vi "Control.vi"() -> ()   [LabVIEW 2021]
uses:
  <vilib>/Utility/error.llb/DialogType.ctl
  <vilib>/DAQmx/write.llb/DAQmx Write (Digital U8 1Chan 1Samp).vi
  <vilib>/DAQmx/read.llb/DAQmx Read (Analog 1D Wfm NChan 1Samp).vi
  <vilib>/DAQmx/write.llb/DAQmx Write (Analog DBL 1Chan 1Samp).vi
  <vilib>/DAQmx/create/channels.llb/DAQmx Create Channel (AO-Voltage-Basic).vi
  <vilib>/DAQmx/create/channels.llb/DAQmx Create Channel (AI-Voltage-Basic).vi
  <vilib>/DAQmx/create/channels.llb/DAQmx Create Channel (DO-Digital Output).vi
  <vilib>/DAQmx/miscellaneous.llb/DAQmx Fill In Error Info.vi
  <vilib>/Utility/file.llb/Read Delimited Spreadsheet (string).vi
  <vilib>/addons/control/pid/pid.llb/PID (DBL).vi
  <vilib>/Utility/file.llb/Write Delimited Spreadsheet (string).vi
  <vilib>/Analysis/NI_AALBase.lvlib
  <vilib>/addons/control/pid/NI_PID_pid.lvlib
panel:
  out "Duración real":dbl
  out "Señal de error":waveform(dbl)(graph)
  out "Señal de control":waveform(dbl)(graph)
  in  "Offset":dbl=0.0001012992 format="%.6e"
  in  "Amplitud":dbl=0.01 format="%.6e"
  out "Señal de realimentación":waveform(dbl)(graph)
  in  "n":dbl=-0.05522872 format="%.6e"
  in  "m":dbl=0.01426491 format="%_6e"
  out "Archivo a generar":string
  out "Experimento Nº":i16=1
  in  "Grabar":bool
  out "Salida sensor de curvatura":waveform(dbl)(graph)
  out "Salida sensor de presión":waveform(dbl)(graph)
  in  "Válvula":bool
  in  "stop":bool
  out "Consigna":waveform(dbl)(graph)
  in  "Comenzar":bool
  in  "Ciclo de trabajo":dbl=1.0 format="%#_2f"
  in  "f1":dbl=10.0 format="%.2f"
  in  "Info. muestreo":cluster{"Fs":dbl, "t":dbl}={"Fs"=100.0, "t"=10.0} {"Fs" format="%.2p"}
  in  "Fase":dbl format="%.2f"
  in  "f0":dbl=10.0 format="%.2f"
  in  "Señal":u16(ring)=2 items=["Senoidal", "Chirp", "Escalón"]
  out "Salida regulador de presión":waveform(dbl)(graph)
  in  "Parar":bool
  # "+"
  # "ACTUADOR"
  # "-"
  # "Calibración sensor"
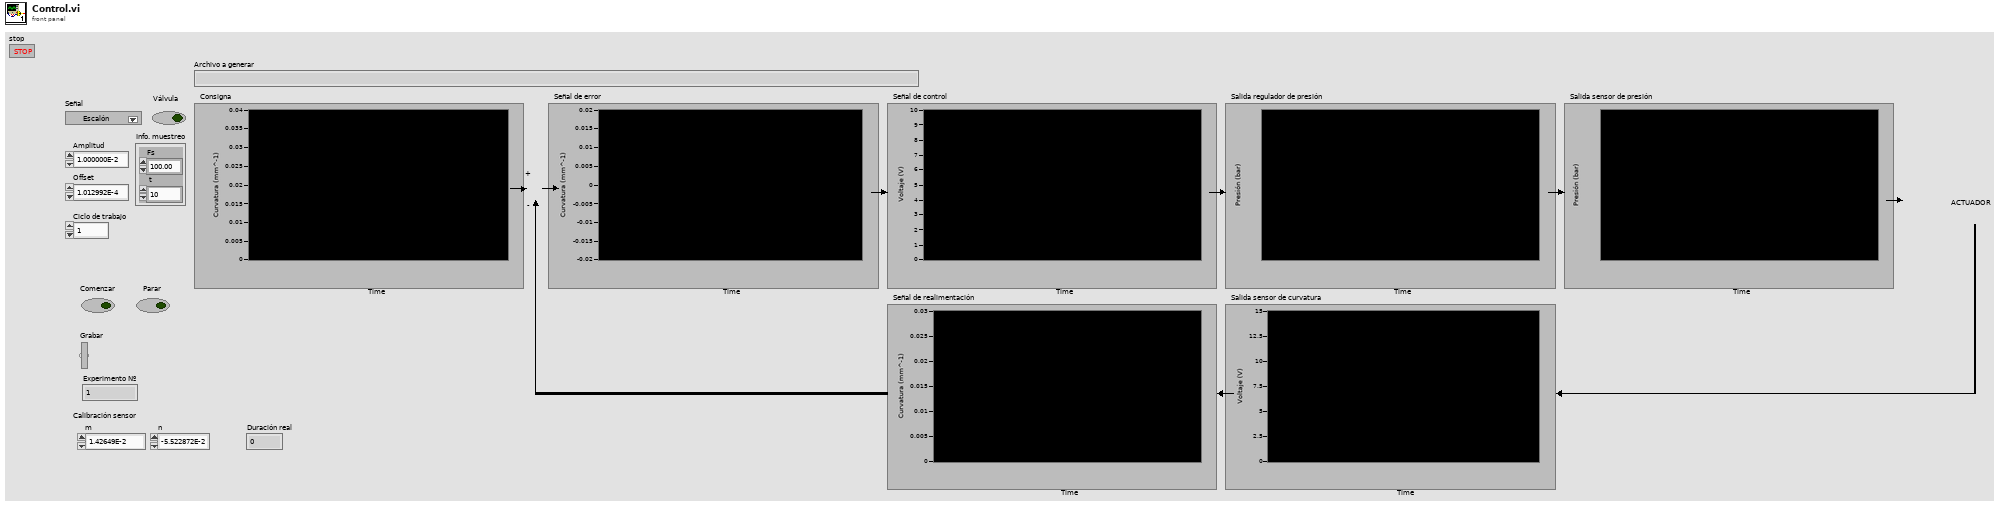
[diagram p1: front panel]
types:
  T1 = cluster{"proportional gain (Kc)":dbl, "integral time (Ti, min)":dbl, "derivative time (Td, min)":dbl}
  T2 = typedef "DialogType.ctl" = u16
  T3 = typedef "NI_Matrix.lvlib/RealMatrix.ctl" = dbl[][]
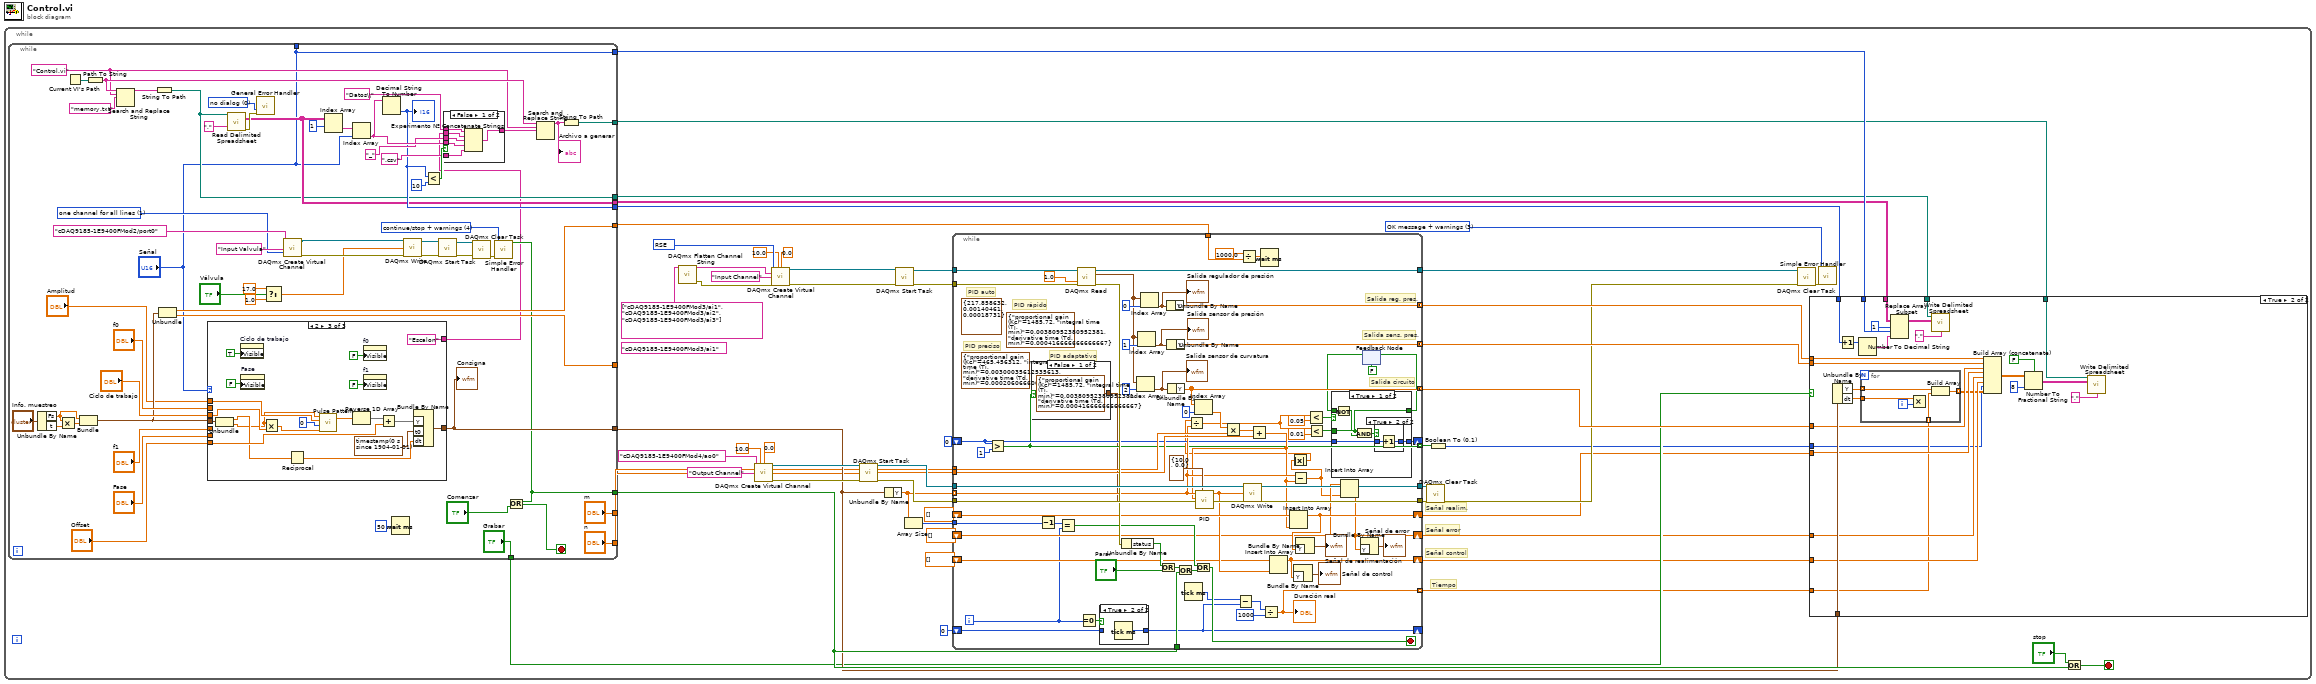
[diagram p0: block diagram]
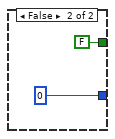
[diagram p4: hidden frame]
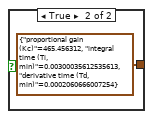
[diagram p5: hidden frame]
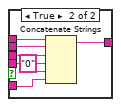
[diagram p7: hidden frame]
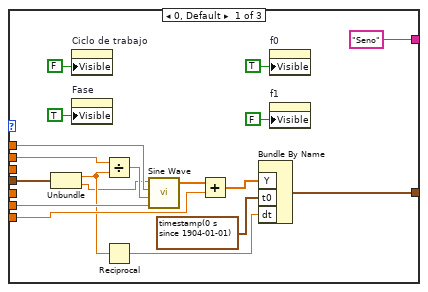
[diagram p8: hidden frame]
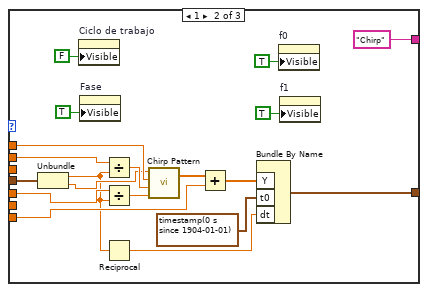
[diagram p9: hidden frame]
diagram:
  n1 = while {
    stop <- w47 stop-if-true
    w49 = T2 3 items=["no dialog", "OK message", "continue or stop message", "OK message + warnings", "continue/stop + warnings"] ("type of dialog (OK msg:1)")
    w45 = 10083 items=["Default"=-1, "RSE"=10083, "NRSE"=10078, "Differential"=10106, "Pseudodifferential"=12529] ("input terminal configuration")
    (unwired) tag "cDAQ9185-1E9400FMod3/ai1" ("physical channels")
    # "Tiempo"
    # "Señal error"
    # "Señal realim."
    # "Señal control"
    n2 = while {
      tunnel: [w222] -> w30
      tunnel: [w229] -> w32
      tunnel: [w223] -> _
      tunnel: [w203] -> w40
      tunnel: ["Señal"] -> _
      tunnel: [w184] -> w28
      tunnel: [w183] -> w27
      tunnel: [w182] -> w26
      tunnel: ["Señal"] -> w29
      tunnel: [w179] -> w25
      tunnel: ["Grabar"] -> w24
      tunnel: ["m"] -> w23
      tunnel: ["n"] -> w22
      stop <- w213 stop-if-true
      w189 = T2 0 items=["no dialog", "OK message", "continue or stop message", "OK message + warnings", "continue/stop + warnings"] ("type of dialog (OK msg:1)")
      w186 = "Control.vi" ("substring (\"\")")
      w208 = 1 items=["one channel for each line", "one channel for all lines"] ("line grouping")
      w220 = T2 4 items=["no dialog", "OK message", "continue or stop message", "OK message + warnings", "continue/stop + warnings"] ("type of dialog (OK msg:1)")
      n3 = Unbundle By Name("Info. muestreo") -> ("Fs"=w225:dbl, "t"=w227:dbl)
      n4 = Multiply(x=w225, y=w227) -> (x*y=w226:dbl)
      n5 = Current VI's Path() -> (path=w194:path)
      n6 = Bundle("Fs"=w225, w226) -> (w224:cluster{"Fs":dbl, dbl})  [unwired: 1 in]
      n7 = Path To String(path=w194) -> (string=w195:string)
      n8 = Search and Replace String(input string=w195, search string=w186, replace string="memory.txt" ("replace string (\"\")")) -> (result string=w196:string)  [unwired: 5 in, 3 out]
      n9 = String To Path(string=w196) -> (path=w182:path)
      n10 = Unbundle(w224) -> ("Fs"=w222:dbl, w223:dbl)
      n11 = case shown="2" "Señal" {
        tunnel: [w261 w273 w301] -> w229
        tunnel: "f0" -> [w259 w279 _]
        tunnel: "Amplitud" -> [w257 w283 w297]
        tunnel: "Fase" -> [w255 _ _]
        tunnel: w224 -> [w254 w272 w291]
        tunnel: "f1" -> [_ w280 _]
        tunnel: "Offset" -> [w260 w281 w293]
        tunnel: "Ciclo de trabajo" -> [_ _ w299]
        tunnel: ["Seno" "Chirp" "Escalon"] -> w180
        frame 0, Default {
          n12 = Unbundle(w254) -> ("Fs"=w253:dbl, w252:dbl)
          n13 = property on="Ciclo de trabajo" class="DigNum (strict)"("Visible"=FALSE) -> ()  [unwired: 2 in, 2 out]
          n14 = property on="Fase" class="DigNum (strict)"("Visible"=TRUE) -> ()  [unwired: 2 in, 2 out]
          n15 = Divide(x=w259, y=w253) -> (x/y=w256:dbl)
          n16 = Reciprocal(x=w253) -> (1/x=w263:dbl)
          n17 = call <vilib>:"Sine Wave.vi"("samples"=w252, "amplitude"=w257, "frequency"=w256, "phase in"=w255) -> ("sine wave"=w258:dbl[])  [unwired: 1 in, 2 out]
          n18 = Add(x=w258, y=w260) -> (x+y=w262:dbl[])
          n19 = Bundle By Name("Y"=w262, "t0"=timestamp(0 s since 1904-01-01), "dt"=w263) -> (w261:waveform(dbl))  [unwired: 1 in]
          n20 = property on="f0" class="DigNum (strict)"("Visible"=TRUE) -> ()  [unwired: 2 in, 2 out]
          n21 = property on="f1" class="DigNum (strict)"("Visible"=FALSE) -> ()  [unwired: 2 in, 2 out]
        }
        frame 1 {
          n22 = Unbundle(w272) -> ("Fs"=w270:dbl, w271:dbl)
          n23 = property on="Ciclo de trabajo" class="DigNum (strict)"("Visible"=FALSE) -> ()  [unwired: 2 in, 2 out]
          n24 = property on="Fase" class="DigNum (strict)"("Visible"=TRUE) -> ()  [unwired: 2 in, 2 out]
          n25 = Divide(x=w279, y=w270) -> (x/y=w278:dbl)
          n26 = Divide(x=w280, y=w270) -> (x/y=w277:dbl)
          n27 = Reciprocal(x=w270) -> (1/x=w275:dbl)
          n28 = call <vilib>:"Chirp Pattern.vi"("f2"=w277, "f1"=w278, "amplitude"=w283, "samples"=w271) -> ("Chirp Pattern"=w282:dbl[])  [unwired: 1 out]
          n29 = Add(x=w282, y=w281) -> (x+y=w274:dbl[])
          n30 = Bundle By Name("Y"=w274, "t0"=timestamp(0 s since 1904-01-01), "dt"=w275) -> (w273:waveform(dbl))  [unwired: 1 in]
          n31 = property on="f0" class="DigNum (strict)"("Visible"=TRUE) -> ()  [unwired: 2 in, 2 out]
          n32 = property on="f1" class="DigNum (strict)"("Visible"=TRUE) -> ()  [unwired: 2 in, 2 out]
        }
        frame 2 {
          n33 = Unbundle(w291) -> ("Fs"=w290:dbl, w289:dbl)
          n34 = property on="Ciclo de trabajo" class="DigNum (strict)"("Visible"=TRUE) -> ()  [unwired: 2 in, 2 out]
          n35 = property on="Fase" class="DigNum (strict)"("Visible"=FALSE) -> ()  [unwired: 2 in, 2 out]
          n36 = Multiply(x=w289, y=w299) -> (x*y=w298:dbl)
          n37 = Reciprocal(x=w290) -> (1/x=w300:dbl)
          n38 = call <vilib>:"Pulse Pattern.vi"("width"=w298, "delay"=0, "amplitude"=w297, "samples"=w289) -> ("Pulse Pattern"=w295:dbl[])  [unwired: 1 out]
          n39 = Reverse 1D Array(array=w295) -> (reversed array=w294:dbl[])
          n40 = property on="f0" class="DigNum (strict)"("Visible"=FALSE) -> ()  [unwired: 2 in, 2 out]
          n41 = property on="f1" class="DigNum (strict)"("Visible"=FALSE) -> ()  [unwired: 2 in, 2 out]
          n42 = Add(x=w294, y=w293) -> (x+y=w292:dbl[])
          n43 = Bundle By Name("Y"=w292, "t0"=timestamp(0 s since 1904-01-01), "dt"=w300) -> (w301:waveform(dbl))  [unwired: 1 in]
        }
      }
      "Consigna" <- w229
      n44 = call-poly <vilib>:"Read Delimited Spreadsheet.vi"("file path (dialog if empty)"=w182, "delimiter (\\t)"="," ("delimiter (\\t)")) -> ("all rows"=w183:string[][], "error out"=w201:errorcluster)  [unwired: 8 in, 4 out]
      n45 = call <vilib>:"General Error Handler.vi"("type of dialog (OK msg:1)"=w189, "error in (no error)"=w201) -> ()  [unwired: 9 in, 5 out]
      n46 = Select(t=17.0, s="Válvula", f=1.0) -> (s? t:f=w206:dbl)
      n47 = call-poly <vilib>:"DAQmx Create Virtual Channel.vi"("lines"=tag "cDAQ9185-1E9400FMod2/port0", "name to assign"="Input Valvula", "line grouping"=w208) -> ("task out"=w211:refnum<k21>, "error out"=w212:errorcluster)  [unwired: 11 in]
      n48 = Index Array(array=w183, index (row)=1) -> (element=w197:string[])  [unwired: 1 in]
      n49 = Index Array(array=w197, index="Señal") -> (element=w200:string)
      n50 = Decimal String To Number(string=w200) -> (number=w184:i32)  [unwired: 2 in, 1 out]
      "Experimento Nº" <- w184
      n51 = Wait (ms)(milliseconds to wait=u32 50) -> ()  [unwired: 1 out]
      n52 = call-poly <vilib>:"DAQmx Write.vi"("task/channels in"=w211, "data"=w206, "error in"=w212) -> ("task out"=w215:refnum<k21>, "error out"=w214:errorcluster)  [unwired: 10 in, 1 out]
      n53 = Less?(x=w184, y=10) -> (x < y?=w202:bool)
      n54 = call <vilib>:"DAQmx Start Task.vi"("task/channels in"=w215, "error in"=w214) -> ("task out"=w216:refnum<k21>, "error out"=w217:errorcluster)  [unwired: 12 in]
      n55 = case shown="False" w202 {
        tunnel: "_" ("string") -> [w237 w246]
        tunnel: "Datos\\" ("replace string (\"\")") -> [w238 w245]
        tunnel: [w239 w244] -> w198
        tunnel: ".csv" ("string") -> [w235 w243]
        tunnel: w200 -> [w236 w242]
        tunnel: w180 -> [w234 w240]
        frame False {
          n56 = Concatenate Strings(w238, w234, w237, w236, w235) -> (w239:string)
        }
        frame True {
          n57 = Concatenate Strings(w245, w240, w246, "0" ("string"), w242, w243) -> (w244:string)
        }
      }
      n58 = call <vilib>:"DAQmx Clear Task.vi"("task in"=w216, "error in"=w217) -> ("error out"=w221:errorcluster)  [unwired: 13 in]
      n59 = call <vilib>:"Simple Error Handler.vi"("type of dialog (OK msg:1)"=w220, "error in (no error)"=w221) -> ("error?"=w203:bool)  [unwired: 3 in, 4 out]
      n60 = Or(x=w203, y="Comenzar") -> (x .or. y?=w213:bool)
      n61 = Search and Replace String(input string=w195, search string=w186, replace string=w198) -> (result string=w199:string)  [unwired: 5 in, 3 out]
      "Archivo a generar" <- w199
      n62 = String To Path(string=w199) -> (path=w179:path)
    }
    n63 = call <vilib>:"DAQmx Flatten Channel String.vi"("names in"=string[] ["cDAQ9185-1E9400FMod3/ai1", "cDAQ9185-1E9400FMod3/ai2", "cDAQ9185-1E9400FMod3/ai3"]) -> ("names out"=w44:string, "error out"=w42:errorcluster)  [unwired: 13 in]
    n64 = call-poly <vilib>:"DAQmx Create Virtual Channel.vi"("maximum value"=10.0, "minimum value"=0.0, "physical channels"=tag "cDAQ9185-1E9400FMod4/ao0", "name to assign"="Output Channel") -> ("task out"=w34:refnum<k21>, "error out"=w33:errorcluster)  [unwired: 10 in]
    n65 = call-poly <vilib>:"DAQmx Create Virtual Channel.vi"("maximum value"=10.0, "minimum value"=0.0, "input terminal configuration"=w45, "physical channels"=w44, "name to assign"="Input Channel", "error in"=w42) -> ("task out"=w36:refnum<k21>, "error out"=w35:errorcluster)  [unwired: 8 in]
    n66 = call <vilib>:"DAQmx Start Task.vi"("task/channels in"=w34, "error in"=w33) -> ("task out"=w52:refnum<k21>, "error out"=w41:errorcluster)  [unwired: 12 in]
    n67 = Unbundle By Name(w32) -> ("Y"=w8:dbl[])
    n68 = call <vilib>:"DAQmx Start Task.vi"("task/channels in"=w36, "error in"=w35) -> ("task out"=w12:refnum<k21>, "error out"=w9:errorcluster)  [unwired: 12 in]
    n69 = Array Size(array=w8) -> (size(s)=w7:i32)
    n70 = while {
      tunnel: w12 -> [w126]
      tunnel: w9 -> [w125]
      tunnel: w52 -> [w111]
      tunnel: [w119] -> w51
      tunnel: [w122] -> w39 mode=concatenating
      tunnel: [w106] -> w38 mode=concatenating
      tunnel: [w109] -> w11
      tunnel: w41 -> [w110]
      tunnel: [w108] -> w10
      tunnel: [w97] -> w37 mode=concatenating
      tunnel: w40 -> [w114]
      tunnel: w8 -> [w75] mode=indexing
      tunnel: w30 -> [w104]
      tunnel: w7 -> [w103]
      tunnel: w23 -> [w95]
      tunnel: w22 -> [w93]
      shift-right: [w90] -> w21
      shift-left: dbl[] [] -> [w92]
      shift-right: [w86] -> w19
      shift-left: dbl[] [] -> [w87]
      shift-right: [w82] -> w18
      shift-left: dbl[] [] -> [w84]
      tunnel: [w76] -> w14 mode=indexing
      shift-right: [w71] -> _
      shift-left: 0 -> [w70]
      tunnel: [w56] -> w2 mode=indexing
      shift-right: [w57] -> _
      shift-left: u32 0 ("millisecond timer value") -> [w58]
      i -> [w59]
      stop <- w99 stop-if-true
      (unwired) T1 {"proportional gain (Kc)"=1485.72, "integral time (Ti, min)"=0.00380952380952381, "derivative time (Td, min)"=0.000416666666666667} ("PID gains")
      (unwired) T1 {"proportional gain (Kc)"=465.456312, "integral time (Ti, min)"=0.00300035612535613, "derivative time (Td, min)"=0.0002060666007254} ("PID gains")
      (unwired) T1 {"proportional gain (Kc)"=217.858632, "integral time (Ti, min)"=0.00140461, "derivative time (Td, min)"=0.00018731} ("PID gains")
      # "PID adaptativo"
      # "PID rápido"
      # "PID preciso"
      # "PID auto"
      # "Salida circuito"
      # "Salida sens. pres."
      # "Salida reg. pres."
      n71 = Greater?(x=w70, y=1) -> (0:w56:bool)
      n72 = case shown="False" w56 {
        tunnel: [T1 {"proportional gain (Kc)"=1485.72, "integral time (Ti, min)"=0.00380952380952381, "derivative time (Td, min)"=0.000416666666666667} ("PID gains") T1 {"proportional gain (Kc)"=465.456312, "integral time (Ti, min)"=0.00300035612535613, "derivative time (Td, min)"=0.0002060666007254} ("PID gains")] -> w55
        frame False {
        }
        frame True {
        }
      }
      n73 = Decrement(x=w103) -> (x-1=w102:i32)
      n74 = Equal?(x=w102, y=w59) -> (x = y?=w100:bool)
      n75 = call-poly <vilib>:"DAQmx Read.vi"("task/channels in"=w126, "timeout"=1.0, "error in"=w125) -> ("task out"=w119:refnum<k21>, "data"=w116:waveform(dbl)[], "error out"=w107:errorcluster)  [unwired: 10 in]
      n76 = Equal To 0?(x=w59) -> (x = 0?=w60:bool)
      n77 = case shown="True" w60 {
        tunnel: [w127 w128] -> w57
        tunnel: w58 -> [w127 _]
        frame False {
        }
        frame True {
          n78 = Tick Count (ms)() -> (millisecond timer value=w128:u32)
        }
      }
      n79 = Unbundle By Name(w107) -> ("status"=w118:bool)
      n80 = Index Array(array=w116, index=2) -> (element=w96:waveform(dbl))
      "Salida sensor de curvatura" <- w96
      n81 = Index Array(array=w116, index=1) -> (element=w112:waveform(dbl))
      "Salida sensor de presión" <- w112
      n82 = Index Array(array=w116, index=0) -> (element=w113:waveform(dbl))
      "Salida regulador de presión" <- w113
      n83 = Or(x=w118, y="Parar") -> (x .or. y?=w115:bool)
      n84 = Unbundle By Name(w113) -> ("Y"=w122:dbl[])
      n85 = Unbundle By Name(w112) -> ("Y"=w106:dbl[])
      n86 = Unbundle By Name(w96) -> ("Y"=w97:dbl[])
      n87 = Or(x=w115, y=w114) -> (x .or. y?=w101:bool)
      n88 = Tick Count (ms)() -> (millisecond timer value=w80:u32)
      n89 = Or(x=w100, y=w101) -> (x .or. y?=w99:bool)
      n90 = Index Array(array=w97, index=0) -> (element=w81:dbl)
      n91 = Multiply(x=w81, y=w95) -> (x*y=w94:dbl)
      n92 = Subtract(x=w80, y=w57) -> (x-y=w77:u32)
      n93 = Divide(x=1000.0, y=w104) -> (x/y=w79:dbl)
      n94 = Add(x=w94, y=w93) -> (x+y=w74:dbl)
      n95 = call-poly <vilib>:"PID.vi"("output range"=cluster{"output high":dbl, "output low":dbl} {"output high"=10.0, "output low"=0.0}, "PID gains"=w55, "process variable"=w74, "setpoint"=w75) -> ("output"=w88:dbl)  [unwired: 6 in, 1 out]
      n96 = call-poly <vilib>:"DAQmx Write.vi"("task/channels in"=w111, "data"=w88, "error in"=w110) -> ("task out"=w109:refnum<k21>, "error out"=w108:errorcluster)  [unwired: 10 in, 1 out]
      n97 = Wait (ms)(milliseconds to wait=w79) -> ()  [unwired: 1 out]
      n98 = Divide(x=w77, y=u32 1000) -> (x/y=w76:dbl)
      "Duración real" <- w76
      n99 = Insert Into Array(array=w87, new element=w88) -> (w86:dbl[])  [unwired: 1 in]
      n100 = Insert Into Array(array=w92, new element=w74) -> (w90:dbl[])  [unwired: 1 in]
      n101 = Subtract(x=w75, y=w74) -> (x-y=w63:dbl)
      n102 = Absolute Value(x=w63) -> (abs(x)=w62:dbl)
      n103 = Divide(x=w62, y=w75) -> (x/y=w61:dbl)
      n104 = Bundle By Name("Y"=w86) -> (→"Señal de control":waveform(dbl))  [unwired: 1 in]
      n105 = Bundle By Name("Y"=w90) -> (→"Señal de realimentación":waveform(dbl))  [unwired: 1 in]
      n106 = Less?(x=w61, y=0.05) -> (x < y?=w73:bool)
      n107 = Less?(x=w61, y=0.01) -> (x < y?=w64:bool)
      n108 = Insert Into Array(array=w84, new element=w63) -> (w82:dbl[])  [unwired: 1 in]
      n109 = Bundle By Name("Y"=w82) -> (→"Señal de error":waveform(dbl))  [unwired: 1 in]
      n110 = feedback #1(FALSE) -> (w68:bool)
      n111 = case shown="True" w73 {
        tunnel: [w133 0] -> w71
        tunnel: w70 -> [w134 _]
        tunnel: w64 -> [w131 _]
        tunnel: [w131 FALSE] -> w66
        tunnel: w68 -> [w130 _]
        frame True {
          n112 = Not(x=w130) -> (.not. x?=w129:bool)
          n113 = And(x=w131, y=w129) -> (x .and. y?=w132:bool)
          n114 = case shown="True" w132 {
            tunnel: w134 -> [w135 w137]
            tunnel: [w135 w136] -> w133
            frame False {
            }
            frame True {
              n115 = Increment(x=w137) -> (x+1=w136:i32)
            }
          }
        }
        frame False {
        }
      }
      n116 = feedback-in #1(w66) -> ()
    }
    n117 = call <vilib>:"DAQmx Clear Task.vi"("task in"=w11, "error in"=w10) -> ("error out"=w31:errorcluster)  [unwired: 13 in]
    n118 = Boolean To (0,1)(Boolean=w2) -> (0, 1=w13:i16[])
    n119 = call <vilib>:"DAQmx Clear Task.vi"("task in"=w51, "error in"=w31) -> ("error out"=w50:errorcluster)  [unwired: 13 in]
    n120 = case shown="True" w24 {
      tunnel: w32 -> [_ w167]
      tunnel: w39 -> [_ w166]
      tunnel: w38 -> [_ w165]
      tunnel: w37 -> [_ w164]
      tunnel: w29 -> [_ w153]
      tunnel: w28 -> [_ w152]
      tunnel: w27 -> [_ w150]
      tunnel: w26 -> [_ w151]
      tunnel: w25 -> [_ w148]
      tunnel: w21 -> [_ w147]
      tunnel: w19 -> [_ w145]
      tunnel: w18 -> [_ w146]
      tunnel: w14 -> [_ w144]
      tunnel: w13 -> [_ w142]
      frame False {
      }
      frame True {
        n121 = Unbundle By Name(w167) -> ("Y"=w168:dbl[], "dt"=w154:dbl)
        n122 = Increment(x=w152) -> (x+1=w158:i32)
        n123 = Number To Decimal String(number=w158) -> (decimal integer string=w155:string)  [unwired: 1 in]
        n124 = for {
          tunnel: w168 -> [w172] mode=indexing
          tunnel: [w171] -> w143 mode=indexing
          tunnel: w154 -> [w170]
          tunnel: w144 -> [w169] mode=indexing
          i -> [w173]
          n125 = Multiply(x=w170, y=w173) -> ()  [unwired: 1 out]
          n126 = Build Array(w172, w169) -> (w171:dbl[])
        }
        n127 = Replace Array Subset(array=w150, new element=w155, index (row)=1, index (col)=w153) -> (w149:string[][])
        n128 = call-poly <vilib>:"Write Delimited Spreadsheet.vi"("file path (dialog if empty)"=w151, "2D data"=w149, "delimiter (\\t)"="," ("delimiter (\\t)")) -> ()  [unwired: 11 in, 2 out]
        n129 = Build Array (concatenate)(w166, w165, w164, w147, w146, w145, w142, w143) -> (w159:T3)
        n130 = Number To Fractional String(use system decimal point (T)=FALSE, number=w159, precision (6)=i16 8) -> (F-format string=w160:string[][])  [unwired: 1 in]
        n131 = call-poly <vilib>:"Write Delimited Spreadsheet.vi"("file path (dialog if empty)"=w148, "2D data"=w160, "delimiter (\\t)"="," ("delimiter (\\t)")) -> ()  [unwired: 11 in, 2 out]
      }
    }
    n132 = call <vilib>:"Simple Error Handler.vi"("type of dialog (OK msg:1)"=w49, "error in (no error)"=w50) -> ()  [unwired: 3 in, 5 out]
    n133 = Or(x="stop", y=w40) -> (x .or. y?=w47:bool)
  }
